vi "split path at final key.vi"(11 "string":string) -> (2 "String":string, 3 "String 2":string)   [LabVIEW 2016, in "JSON Value.lvclass"]
uses:
  JSON Value.lvclass
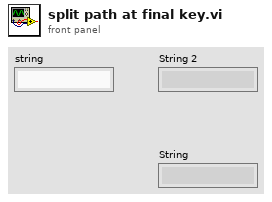
[diagram p1: front panel]
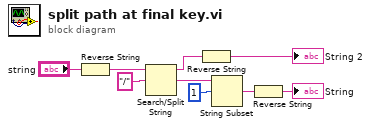
[diagram p0: block diagram]
diagram:
  n1 = Reverse String(1:"string") -> (0:w6:string)
  n2 = Search/Split String(string=w6, search string/char (-)="/") -> (substring before match=w7:string, match + rest of string=w3:string)  [unwired: 1 in, 1 out]
  n3 = Reverse String(1:w7) -> (0:→"String 2":string)
  n4 = String Subset(string=w3, offset (0)=1) -> (substring=w2:string)  [unwired: 1 in]
  n5 = Reverse String(1:w2) -> (0:→"String":string)
